vi "proc.util.errorDescriptor.vi"(5 "stepElement":variant, 7 "procElement":variant, 8 "NextState in":cluster{"CMD":T1, "data":variant}={"CMD"=enum."JUMP", "data"=variant}, 11 "error in":errorcluster) -> (0 "nextState out":cluster{"CMD":T1, "data":variant}={"CMD"=enum."JUMP", "data"=variant}, 1 "errorMsg":string, 3 "error out":errorcluster)   [LabVIEW 2024]
uses:
  controls/typeCmdPostStepFunc.ctl
  Polymorphics/variantCtrlStepIoPointer.vi
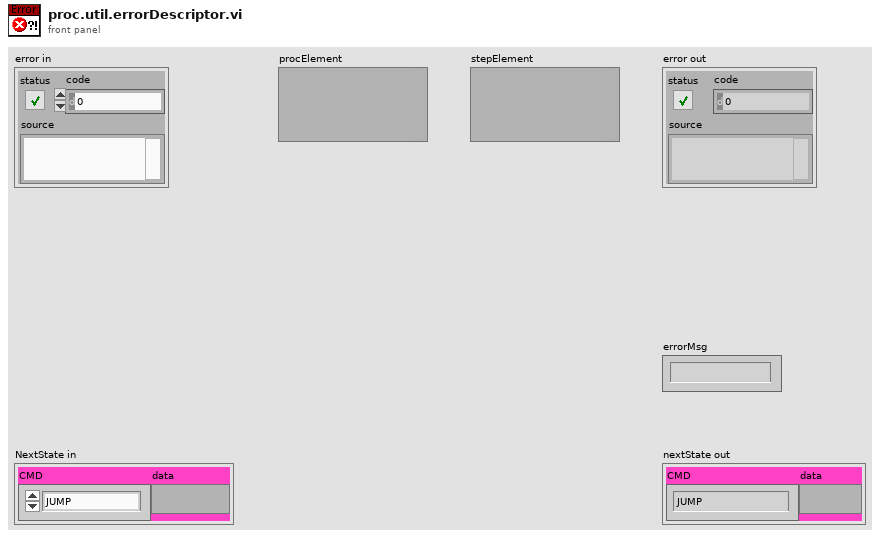
[diagram p1: front panel]
types:
  T1 = typedef "typeCmdPostStepFunc.ctl" = enum16{"NEXT", "PREV", "JUMP", "STAY", "COMPLETE", "ENGCALL.PROC.START", "ENGCALL.PROC.STOP", "ENGCALL.PROC.COMPLETION-CHECK", "ENGCALL.PROC.INIT", "ERROR"}
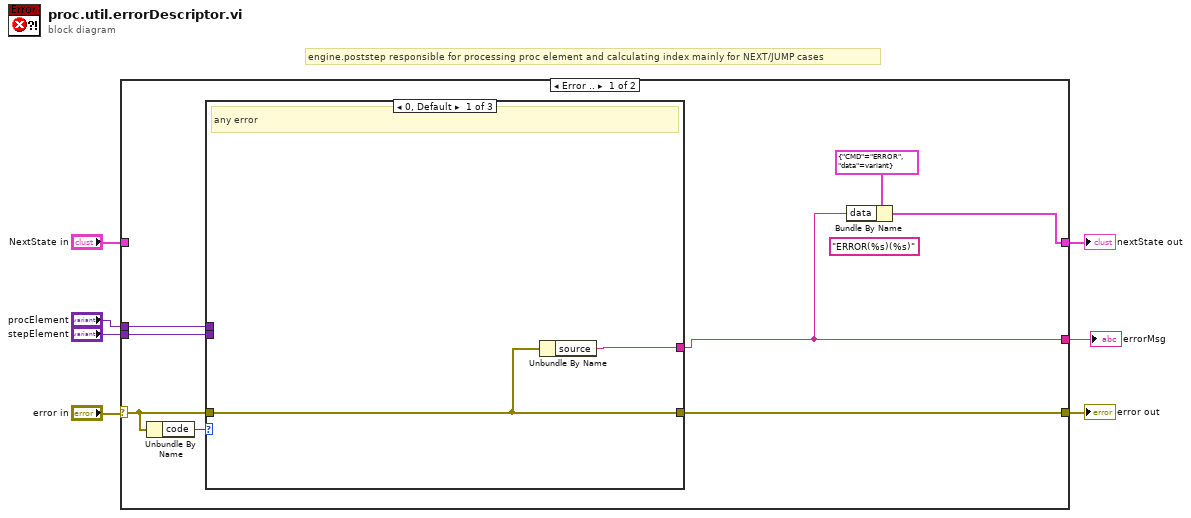
[diagram p0: block diagram]
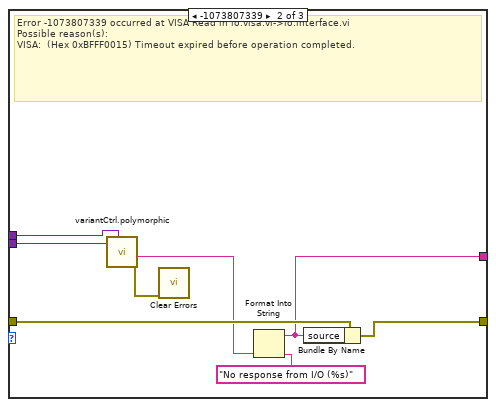
[diagram p2: hidden frame]
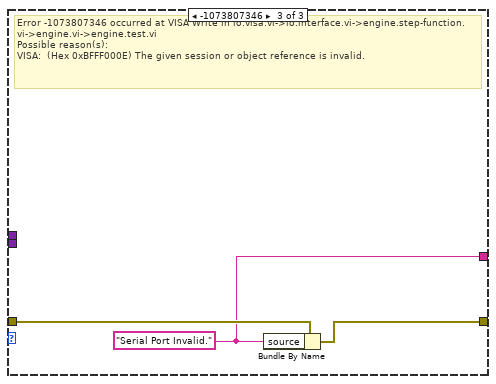
[diagram p3: hidden frame]
diagram:
  # "engine.poststep responsible for processing proc element and calculating index mainly for NEXT/JUMP cases"
  n1 = case shown="Error .." "error in" {
    selector: "error in" -> [w12 w30]
    tunnel: "procElement" -> [w11 _]
    tunnel: "NextState in" -> [_ w29]
    tunnel: [w13 w30] -> w7
    tunnel: [w14 w29] -> w2
    tunnel: "stepElement" -> [w10 _]
    tunnel: [w8 _] -> w1
    frame Error {
      (unwired) "ERROR(%s)(%s)" ("format string")
      n2 = Unbundle By Name(w12) -> ("code"=w15:i32)
      n3 = case shown="0, Default" w15 {
        tunnel: [w17 w24 w27] -> w13
        tunnel: w12 -> [w17 w25 w28]
        tunnel: w11 -> [_ w19 _]
        tunnel: w10 -> [_ w22 _]
        tunnel: [w16 w20 w26] -> w8
        frame 0, Default {
          # "any error"
          n4 = Unbundle By Name(w17) -> ("source"=w16:string)
        }
        frame -1073807339 {
          # "Error -1073807339 occurred at VISA Read in io.visa.vi->io.interface.vi\nPossible reason(s):\nVISA:  (Hex 0xBFFF0015) Timeout expired before operation completed."
          n5 = call-poly "variantCtrl.polymorphic.vi"("procElement"=w19, "StepElement in"=w22) -> ("error out"=w18:errorcluster, "I/O Pointer out"=w21:string)  [unwired: 6 in, 2 out]
          n6 = call <vilib>:"Clear Errors.vi"("error in (no error)"=w18) -> ()  [unwired: 5 in, 2 out]
          n7 = Format Into String(format string="No response from I/O (%s)" ("source"), w21) -> (resulting string=w20:string)  [unwired: 2 in, 1 out]
          n8 = Bundle By Name(cluster=w25, "source"=w20) -> (w24:errorcluster)
        }
        frame -1073807346 {
          w26 = "Serial Port Invalid." ("source")
          # "Error -1073807346 occurred at VISA Write in io.visa.vi->io.interface.vi->engine.step-function.vi->engine.vi->engine.test.vi\nPossible reason(s):\nVISA:  (Hex 0xBFFF000E) The given session or object reference is invalid."
          n9 = Bundle By Name(cluster=w28, "source"=w26) -> (w27:errorcluster)
        }
      }
      n10 = Bundle By Name(cluster=cluster{"CMD":T1, "data":variant} {"CMD"=enum."ERROR", "data"=variant} ("Next State"), "data"=w8) -> (w14:cluster{"CMD":T1, "data":variant})
    }
    frame No Error {
    }
  }
  "error out" <- w7
  "nextState out" <- w2
  "errorMsg" <- w1
